vi "Stop_Test.vi"() -> (3 "Failed?":bool)   [LabVIEW 2017, in "WordManipulationTests.lvlib"]
uses:
  WordManipulationTests.lvlib
  Utilities/WordManipulationLibrary.lvlib
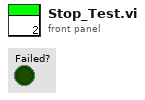
[diagram p1: front panel]
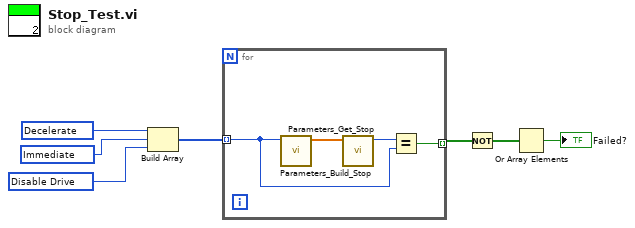
[diagram p0: block diagram]
diagram:
  w5 = 11599970 items=["Decelerate"=11599968, "Immediate"=11599969, "Disable Drive"=11599970] ("Stop Mode")
  w6 = 11599969 items=["Decelerate"=11599968, "Immediate"=11599969, "Disable Drive"=11599970] ("Stop Mode")
  w7 = 11599968 items=["Decelerate"=11599968, "Immediate"=11599969, "Disable Drive"=11599970] ("Stop Mode")
  n1 = Build Array(w7, w6, w5) -> (w4:i32[])
  n2 = for {
    tunnel: w4 -> [w9] mode=indexing
    tunnel: [w8] -> w3 mode=indexing
    n3 = call "Parameters_Build_Stop.vi"("Stop Mode"=w9) -> ("Parameters"=w11:dbl[])  [unwired: 10 in]
    n4 = call "Parameters_Get_Stop.vi"("Parameters"=w11) -> ("Stop Mode"=w10:i32)  [unwired: 10 in]
    n5 = Equal?(x=w10, y=w9) -> (x = y?=w8:bool)
  }
  n6 = Not(x=w3) -> (.not. x?=w2:bool[])
  n7 = Or Array Elements(Boolean array=w2) -> (logical OR=→"Failed?":bool)
